vi "PH_Beamline_Common.set MM1.vi"(2 "CtlRef":refnum<vi>, 3 "State":T1 items=["unknown", "Position I", "Position II", "Position III", "Position IV", "moving"], 4 "no link":bool, 5 "error in (no error)":errorcluster) -> (19 "error out":errorcluster)   [LabVIEW 2014, in "PH_Beamline_Common.lvlib"]
uses:
  PH_Beamline_Common.lvlib
  PH_Motion/PH_4_Pos_Selector/PH_4_Pos_Selector.Position Selector.ctl
  PH_Common/PH_Common.lvlib
  PH_Motion/PH_4_Pos_Selector/PH_4_Pos_Selector.lvlib
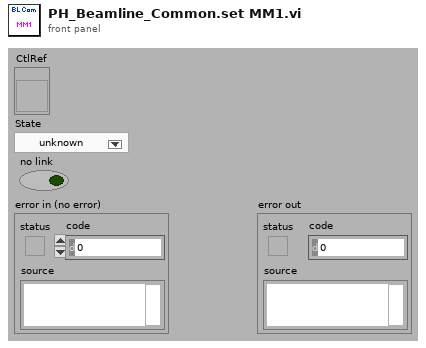
[diagram p1: front panel]
types:
  T1 = typedef "PH_4_Pos_Selector.lvlib/PH_4_Pos_Selector.Position Selector.ctl" = u16
  T2 = cluster{"left":i16, "top":i16, "right":i16, "bottom":i16}
  T3 = cluster{"Width":u16, "Style":enum32{"Solid", "Dash", "Dot", "DashDot", "DashDotDot"}}
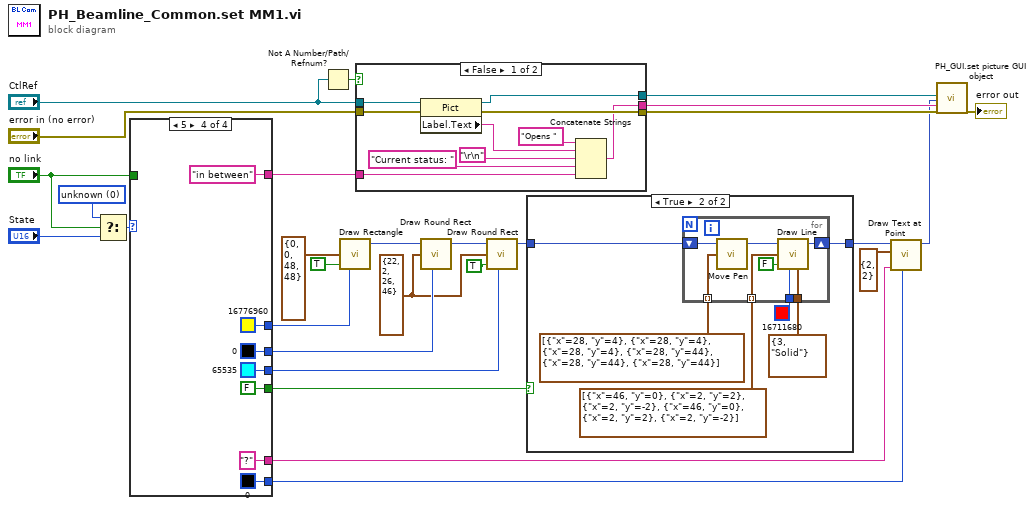
[diagram p0: block diagram]
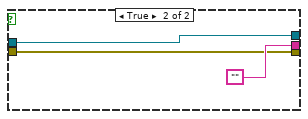
[diagram p3: hidden frame]
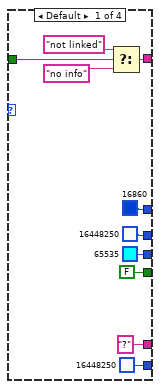
[diagram p4: hidden frame]
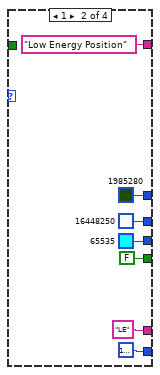
[diagram p5: hidden frame]
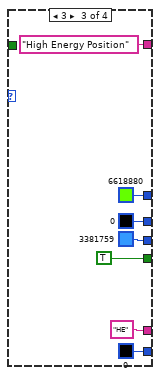
[diagram p6: hidden frame]
diagram:
  w5 = T2 {"left"=22, "top"=2, "right"=26, "bottom"=46} ("rect")
  w7 = T1 0 items=["unknown", "Position I", "Position II", "Position III", "Position IV", "moving"] ("State")
  n1 = Select(t=w7, s="no link", f="State") -> (s? t:f=w19:T1)
  n2 = case shown="5" w19 {
    tunnel: [u32 16860 u32 1985280 u32 6618880 u32 16776960] -> w22
    tunnel: "no link" -> [w34 _ _ _]
    tunnel: [w35 "Low Energy Position" "High Energy Position" "in between"] -> w18
    tunnel: [u32 16448250 u32 16448250 u32 0 u32 0] -> w11
    tunnel: ["?" "LE" "HE" "?"] -> w12
    tunnel: [u32 16448250 u32 16777226 u32 0 u32 0] -> w10
    tunnel: [FALSE FALSE TRUE FALSE] -> w2
    tunnel: [u32 65535 u32 65535 u32 3381759 u32 65535] -> w1
    frame Default {
      n3 = Select(t="not linked", s=w34, f="no info") -> (s? t:f=w35:string)
    }
    frame 1 {
    }
    frame 3 {
    }
    frame 5 {
    }
  }
  n4 = Not A Number/Path/Refnum?(number/path/refnum="CtlRef") -> (NaN/Path/Refnum?=w8:bool)
  n5 = call <vilib>:"Draw Rectangle.vi"("rect"=T2 {"left"=0, "top"=0, "right"=48, "bottom"=48}, "fill?(F)"=TRUE, "color(black)"=w22) -> ("new picture"=w15:picture)  [unwired: 6 in]
  n6 = case shown="False" w8 {
    tunnel: "CtlRef" -> [w65 w72]
    tunnel: "error in (no error)" -> [w64 w70]
    tunnel: [w63 w70] -> w20
    tunnel: w18 -> [w62 _]
    tunnel: [w61 ""] -> w17
    tunnel: [w60 w72] -> w9
    frame False {
      n7 = property class="Pict"(reference=w65, error in=w64) -> (reference out=w60:refnum<vi>, error out=w63:errorcluster, "Label.Text"=w68:string)
      n8 = Concatenate Strings("Opens " ("string"), w68, "\r\n", "Current status: " ("string"), w62) -> (w61:string)
    }
    frame True {
    }
  }
  n9 = call <vilib>:"Draw Round Rect.vi"("picture"=w15, "rect"=w5, "color(black)"=w11) -> ("new picture"=w14:picture)  [unwired: 6 in]
  n10 = call <vilib>:"Draw Round Rect.vi"("picture"=w14, "rect"=w5, "fill?(F)"=TRUE, "color(black)"=w1) -> ("new picture"=w4:picture)  [unwired: 5 in]
  n11 = case shown="True" w2 {
    tunnel: w4 -> [w73 w79]
    tunnel: [w73 w78] -> w3
    frame False {
    }
    frame True {
      n12 = for {
        tunnel: u32 16711680 ("color(black)") -> [w86]
        tunnel: T3 {"Width"=3, "Style"=enum."Solid"} ("pen") -> [w85]
        tunnel: cluster{"x":i16, "y":i16}[] [{"x"=28, "y"=4}, {"x"=28, "y"=4}, {"x"=28, "y"=4}, {"x"=28, "y"=44}, {"x"=28, "y"=44}, {"x"=28, "y"=44}] -> [w81] mode=indexing
        shift-right: [w87] -> w78
        shift-left: w79 -> [w84]
        tunnel: cluster{"x":i16, "y":i16}[] [{"x"=46, "y"=0}, {"x"=2, "y"=2}, {"x"=2, "y"=-2}, {"x"=46, "y"=0}, {"x"=2, "y"=2}, {"x"=2, "y"=-2}] -> [w80] mode=indexing
        n13 = call <vilib>:"Move Pen.vi"("new position"=w81, "picture"=w84) -> ("new picture"=w83:picture)  [unwired: 3 in]
        n14 = call <vilib>:"Draw Line.vi"("picture"=w83, "end point"=w80, "absolute coordinates?(T)"=FALSE, "color(black)"=w86, "pen"=w85) -> ("new picture"=w87:picture)  [unwired: 4 in]
      }
    }
  }
  n15 = call <vilib>:"Draw Text at Point.vi"("text color(black)"=w10, "text"=w12, "origin"=cluster{"x":i16, "y":i16} {"x"=2, "y"=2}, "picture"=w3) -> ("new picture"=w13:picture)  [unwired: 6 in, 1 out]
  n16 = call "PH_GUI.set picture GUI object.vi"("CtlRef"=w9, "Picture"=w13, "Tip Strip (\"\")"=w17, "error in (no error)"=w20) -> ("error out"=→"error out":errorcluster)  [unwired: 15 in]
